vi "Create Mesh Object.vi"(8 "error in (no error)":errorcluster, 10 "Alpha":sgl, 11 "Mesh Object In":refnum<vi>) -> (0 "error out":errorcluster, 3 "Object Ref Out":refnum<vi>)   [LabVIEW 2017, in "3D Plot.lvclass"]
uses:
  <vilib>/Math Plots/3D Math Plots/3D Plot/3D Plot/3D Plot.lvclass
  <vilib>/picture/3D Picture Control/Object/Create Object (name).vi
  <vilib>/picture/3D Picture Control/NI_3D Picture Control.lvlib
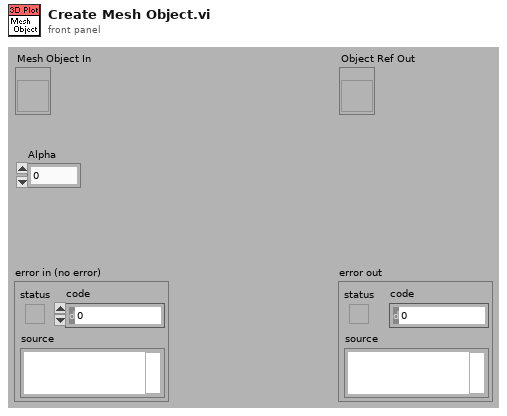
[diagram p1: front panel]
types:
  T1 = enum16{"Inherit Value", "Counterclockwise", "Clockwise"}
  T2 = enum16{"Inherit Material", "Use entire Material", "Ignore Ambient", "Ignore Diffuse", "Ignore Specular", "Ignore Emission", "Ignore Ambient and Diffuse"}
  T3 = enum16{"Normal Bin", "Opaque Bin", "Transparent Bin"}
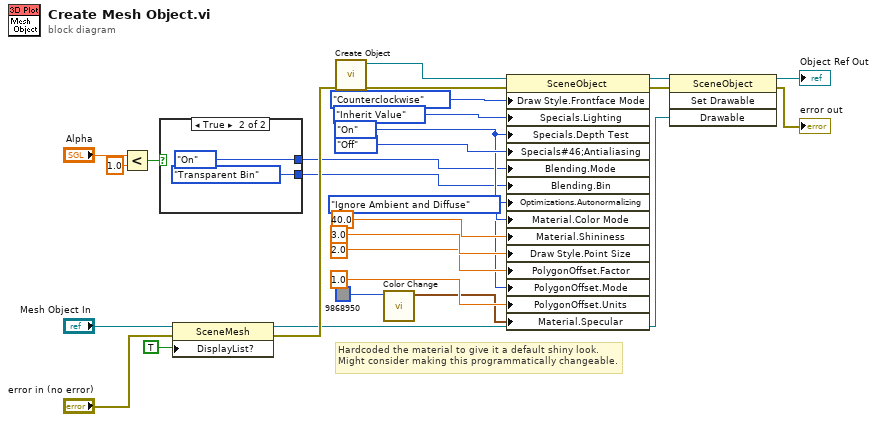
[diagram p0: block diagram]
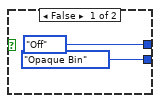
[diagram p2: hidden frame]
diagram:
  w6 = enum16{"Inherit Value", "Off", "On"}."On" ("Specials:Depth Test")
  # "Hardcoded the material to give it a default shiny look.  Might consider making this programmatically changeable."
  n1 = Less?(x="Alpha", y=sgl 1.0) -> (x < y?=w3:bool)
  n2 = case shown="True" w3 {
    tunnel: [T3."Opaque Bin" ("Blending:Bin") T3."Transparent Bin" ("Blending:Bin")] -> w1
    tunnel: [enum16{"Inherit Value", "Off", "On"}."Off" ("Blending:Mode") enum16{"Inherit Value", "Off", "On"}."On" ("Blending:Mode")] -> w2
    frame False {
    }
    frame True {
    }
  }
  n3 = property class="SceneMesh"(reference="Mesh Object In", error in="error in (no error)", "DisplayList?"=TRUE ("Use Display List?")) -> (reference out=w21:refnum<vi>, error out=w23:errorcluster)
  n4 = call-poly <vilib>:"Create Object.vi"("error in (no error)"=w23) -> ("error out"=w18:errorcluster, "Scene:New Object"=w17:refnum<vi>)  [unwired: 9 in]
  n5 = call <vilib>:"Color Change.vi"("Color"=u32 9868950) -> ("RGBA"=w7:cluster{"R":sgl, "G":sgl, "B":sgl, "A":sgl})  [unwired: 1 in, 9 out]
  n6 = property class="SceneObject"(reference=w17, error in=w18, "Draw Style.Frontface Mode"=T1."Counterclockwise" ("Draw Style:Frontface Mode"), "Specials.Lighting"=enum16{"Inherit Value", "Off", "On"}."Inherit Value" ("Specials:Lighting"), "Specials.Depth Test"=w6, "Specials#46;Antialiasing"=enum16{"Inherit Value", "Off", "On"}."Off" ("Specials:Antialiasing"), "Blending.Mode"=w2, "Blending.Bin"=w1, "Optimizations.Autonormalizing"=w6, "Material.Color Mode"=T2."Ignore Ambient and Diffuse" ("Material:Color Mode"), "Material.Shininess"=sgl 40.0 ("Material:Shininess"), "Draw Style.Point Size"=sgl 3.0 ("Draw Style:Point Size"), "PolygonOffset.Factor"=sgl 2.0 ("PolygonOffset:Factor"), "PolygonOffset.Mode"=w6, "PolygonOffset.Units"=sgl 1.0 ("PolygonOffset:Units"), "Material.Specular"=w7) -> (reference out=w25:refnum<vi>, error out=w26:errorcluster)
  n7 = invoke class="SceneObject" method="Set Drawable"(reference=w25, error in=w26, "Drawable"=w21) -> (reference out=→"Object Ref Out":refnum<vi>, error out=→"error out":errorcluster)  [unwired: 1 in, 2 out]
